vi "SVFA FFT Spectrum (Mag-Phase) (1 Ch).vi"(0 "scaled signal [EU]":waveform(dbl), 2 "window":T9=1 items=["None"=0, "Hanning"=1, "Hamming"=2, "Blackman-Harris"=3, "Exact Blackman"=4, "Blackman"=5, "Flat Top"=6, "4 Term B-Harris "=7, "7 Term B-Harris"=8, "Low Sidelobe"=9, "Force"=64, "Exponential"=65, "Blackman Nuttall"=11, "Triangle"=30, "Bartlett-Hanning"=31, "Bohman"=32, "Parzen"=33, "Welch"=34, "Kaiser"=60, "Dolph-Chebyshev"=61, "Gaussian"=62], 4 "view":T7={"dB On (T)"=TRUE, "unwrap phase (F)"=FALSE, "convert to degree (T)"=TRUE}, 5 "error in (no error)":errorcluster, 7 "averaging parameters":T8={"averaging mode"=enum."No averaging", "weighting mode"=enum."Exponential", "number of averages"=10, "linear mode"=enum."One shot"} {"number of averages" min=1 step=1}, 9 "restart averaging (F)":bool) -> (11 "averaging done":bool, 13 "averages completed":dbl, 14 "magnitude [dB EU]":cluster{"f0":dbl, "df":dbl, "magnitude":dbl[]} {"magnitude" format="%.2p"; "df" format="%.2p"; "f0" format="%.2p"}, 15 "magnitude unit label":string, 16 "phase [degrees]":cluster{"f0":dbl, "df":dbl, "phase":dbl[]} {"phase" format="%.2p"; "df" format="%.2p"; "f0" format="%.2p"}, 17 "phase unit label":string, 18 "spectrum info":T1={"channel name"="", "description"="", "x-axis units"=0, "spectral info"={"spectrum type"=enum."Power [Magnitude^2]", "linear/dB"=enum."linear", "window"=0, "window size"=0, "FFT size"=0}, "engineering units"=0, "custom label"="", "dB reference [EU]"=0.0, "peak units"=enum."rms", "weighting filter"=0, "spectral density?"=FALSE, "unit label"="", "spectrum skewed?"=FALSE, "complimentary spectrum units"=enum."none"} {"x-axis units" items=["Time (s)"=0, "Frequency-CB (Hz)"=1, "Frequency-CPB (Hz)"=1248, "Frequency-Arbitrary (Hz)"=2357, "Quefrency (s)"=2, "Revolutions (rev)"=3, "Order"=4, "Speed (RPM)"=11, "Speed (rad/s)"=21, "Index"=65535]; "weighting filter" items=["Linear", "A-weighting", "B-weighting", "C-weighting", "ITU-R 468-4", "Dolby", "CCITT", "C-message", "Wb", "Wc", "Wd", "We", "Wf", "Wh", "Wj", "Wk", "Wm", "AES17 20 kHz lowpass", "AES17 40 kHz lowpass", "AES17 20 kHz highpass", "AES17 40 kHz highpass"]; "dB reference [EU]" format="%.2f"; "engineering units" items=["custom..."=0, "V"=1, "A"=21, "C"=30, "pC"=31, "s"=32, "-"=29, "Pa"=2, "N"=20, "g"=3, "m/s^2"=4, "m/s"=5, "m"=6, "mm/s"=12, "mm"=13, "micron/s"=14, "micron"=15, "in/s^2"=7, "in/s"=8, "in"=9, "mil/s"=10, "mil"=11, "rad/s^2"=16, "rad/s"=17, "rad"=18, "deg/s^2"=26, "deg/s"=27, "deg"=28, "RPM"=22, "cycle/s^2"=23, "Hz"=24, "cycle"=25, "strain"=19]; "spectral info"."window" items=["None "=0, "Hanning"=1, "Hamming"=2, "Blackman-Harris"=3, "Exact Blackman"=4, "Blackman"=5, "Flat Top"=6, "4 Term B-Harris "=7, "7 Term B-Harris"=8, "Low Sidelobe"=9, "Force - Exponential"=10, "Gaussian"=62]}, 19 "error out":errorcluster)   [LabVIEW 2017]
doc: "Computes the Fast Fourier Transform (FFT) spectrum of <B>scaled signal [EU]</B>. This VI returns FFT results as the magnitude and phase of the FFT spectrum. Wire data to the <B>scaled signal [EU]</B> input to determine the polymorphic instance to use or manually select the instance."
uses:
  <vilib>/addons/_NISVFA/_Shared subVIs/Controls/svc_Window.ctl
  <vilib>/addons/_NISVFA/_Shared subVIs/Controls/svc_Spectrum Info.ctl
  <vilib>/addons/_NISVFA/_Shared subVIs/Controls/svc_X-Axis Units.ctl
  <vilib>/addons/_NISVFA/_Shared subVIs/Controls/svc_Spectrum Type.ctl
  <vilib>/addons/_NISVFA/_Shared subVIs/Controls/svc_Engineering Units Text Ring.ctl
  <vilib>/addons/_NISVFA/_Shared subVIs/Controls/svc_Weighting Filter Text Ring.ctl
  <vilib>/addons/_NISVFA/_Shared subVIs/Controls/svc_Complimentary Spectrum Units.ctl
  <vilib>/Analysis/2dsp.llb/Real FFT.vi
  <vilib>/Analysis/2dsp.llb/Power Spectrum (DBL).vi
  <vilib>/addons/_NISVFA/_Shared subVIs/Spectrum Averaging/svfa_No Average Array (complex).vi
  <vilib>/addons/_NISVFA/_Shared subVIs/Spectrum Averaging/svfa_Average Array (complex).vi
  <vilib>/addons/_NISVFA/_Shared subVIs/Spectrum Averaging/svfa_No Average Array (real).vi
  <vilib>/addons/_NISVFA/_Shared subVIs/Spectrum Averaging/svfa_Average Array (real).vi
  <vilib>/addons/_NISVFA/_Shared subVIs/Spectrum Averaging/svfa_Peak Hold Array.vi
  <vilib>/addons/_NISVFA/_Shared subVIs/Windowing/svfa_Scaled Time Domain Window (Array).vi
  <vilib>/addons/_NISVFA/_Shared subVIs/Common/svc_Get SV Channel Info.vi
  <vilib>/addons/_NISVFA/_Shared subVIs/Common/svc_Spectrum Units.vi
  <vilib>/Analysis/4window.llb/Force Window.vi
  <vilib>/Analysis/4window.llb/Force Window (DBL).vi
  <vilib>/Analysis/4window.llb/Exponential Window.vi
  <vilib>/Analysis/4window.llb/Exponential Window (DBL).vi
  <vilib>/addons/_NISVFA/_Shared subVIs/Common/svc_Get Weighting Enum and Labels.vi
  <vilib>/addons/_NISVFA/_Shared subVIs/Common/svc_Unit Label Lexical Class.vi
  <vilib>/addons/_NISVFA/_Shared subVIs/Common/svc_Engineering Units to Unit Label.vi
  <vilib>/addons/_NISVFA/_Shared subVIs/Common/svc_Format Value (DBL).vi
  <vilib>/addons/_NISVFA/_Shared subVIs/Common/svc_Channel Info to Spectrum Info.vi
  <vilib>/addons/_NISVFA/_Shared subVIs/Common/svc_Unit Label to Engineering Units.vi
  <vilib>/Utility/error.llb/Error Cluster From Error Code.vi
  <vilib>/Analysis/0measdsp.llb/Scaled Time Domain Window.vi
  <vilib>/Analysis/0measdsp.llb/Scaled Time Domain Window (DBL).vi
  <vilib>/addons/_NISVFA/_Spectrum Processing/subVIs/svfa_Spectrum Info Window to windowTd Type Def.vi
  <vilib>/addons/_NISVFA/_Shared subVIs/Common/svc_Window Parameters.vi
  <vilib>/addons/_NISVFA/_Shared subVIs/Common/svc_Get Window Info.vi
  <vilib>/Analysis/NI_AALPro.lvlib
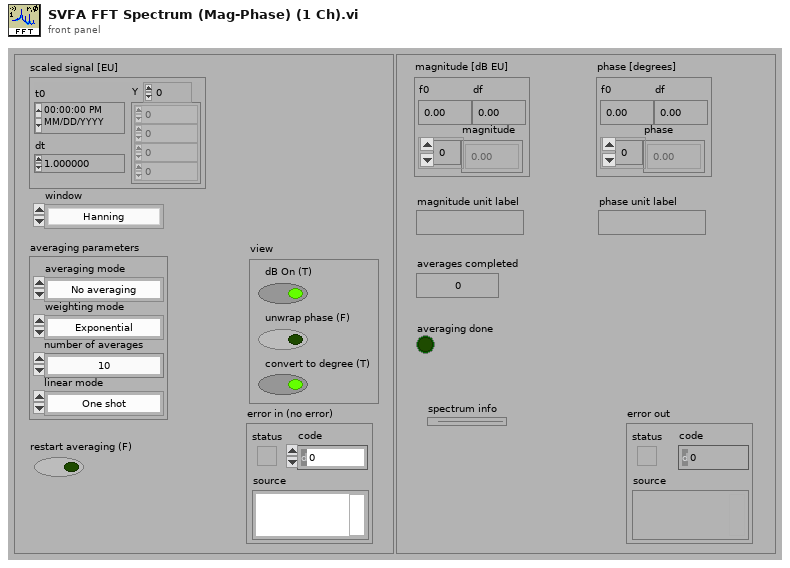
[diagram p1: front panel]
types:
  T1 = typedef "svc_Spectrum Info.ctl" = cluster{"channel name":string, "description":string, "x-axis units":T2, "spectral info":cluster{"spectrum type":T3, "linear/dB":enum16{"linear", "dB"}, "window":u16, "window size":i32, "FFT size":i32}, "engineering units":T4, "custom label":string, "dB reference [EU]":dbl, "peak units":enum16{"rms", "peak", "peak-peak"}, "weighting filter":T5, "spectral density?":bool, "unit label":string, "spectrum skewed?":bool, "complimentary spectrum units":T6}
  T2 = typedef "svc_X-Axis Units.ctl" = u16
  T3 = typedef "svc_Spectrum Type.ctl" = enum16{"FFT Spectrum [complex]", "Amplitude [Magnitude]", "Power [Magnitude^2]", "Cross Spectrum [complex]", "Frequency Response [Complex]"}
  T4 = typedef "svc_Engineering Units Text Ring.ctl" = u16
  T5 = typedef "svc_Weighting Filter Text Ring.ctl" = u16
  T6 = typedef "svc_Complimentary Spectrum Units.ctl" = enum16{"none", "radians", "degrees", "cycles", "imaginary"}
  T7 = cluster{"dB On (T)":bool, "unwrap phase (F)":bool, "convert to degree (T)":bool}
  T8 = cluster{"averaging mode":enum16{"No averaging", "Vector averaging", "RMS averaging", "Peak hold"}, "weighting mode":enum16{"Linear", "Exponential"}, "number of averages":u32, "linear mode":enum16{"One shot", "Auto restart"}}
  T9 = typedef "svc_Window.ctl" = u32
  T10 = cluster{"f0":dbl, "df":dbl, "complex spectrum":cdb[]}
  T11 = enum16{"Restart processing", "Continue processing", "Skip processing"}
  T12 = enum16{"No averaging", "Vector averaging", "RMS averaging", "Peak hold"}
  T13 = cluster{"complex FFT":cdb[], "real FFT":dbl[], "f0":dbl, "df":dbl, "averages completed":dbl, "averaging parameters":cluster{"averaging mode":enum16{"No averaging", "Vector averaging", "RMS averaging", "Peak hold"}, "weighting mode":enum16{"Linear", "Exponential"}, "number of averages":u32, "linear mode":enum16{"One shot", "Auto restart"}}}
  T14 = cluster{"complex FFT":cdb[], "Mag/Real FFT":dbl[], "f0":dbl, "df":dbl, "averages completed":dbl, "averaging parameters":cluster{"averaging mode":enum16{"No averaging", "Vector averaging", "RMS averaging", "Peak hold"}, "weighting mode":enum16{"Linear", "Exponential"}, "number of averages":u32, "linear mode":enum16{"One shot", "Auto restart"}}}
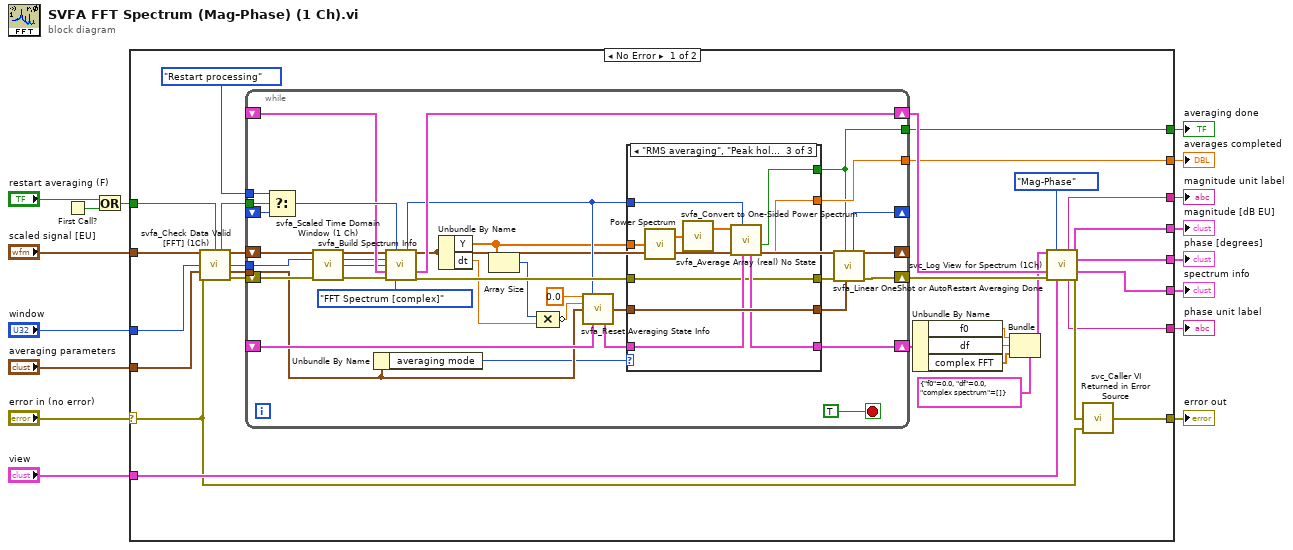
[diagram p0: block diagram]
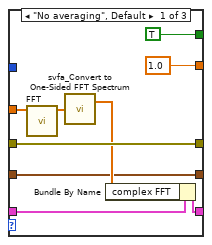
[diagram p2: hidden frame]
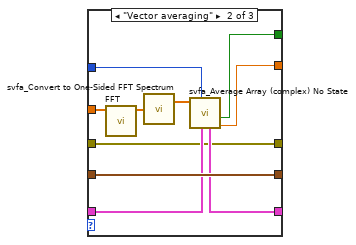
[diagram p3: hidden frame]
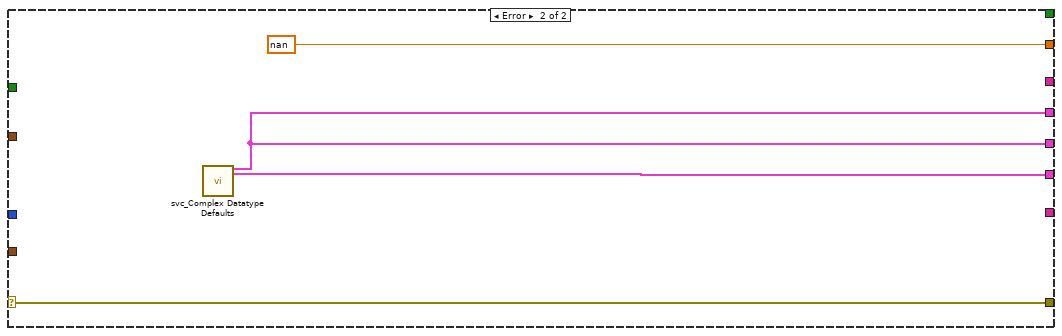
[diagram p4: hidden frame]
diagram:
  n1 = First Call?() -> (First Call?: T/F=w3:bool)
  n2 = Or(x="restart averaging (F)", y=w3) -> (x .or. y?=w1:bool)
  n3 = case shown="No Error" "error in (no error)" {
    selector: "error in (no error)" -> [w18 w114]
    tunnel: [w21 w111] -> w4
    tunnel: "window" -> [w29 _]
    tunnel: "averaging parameters" -> [w30 _]
    tunnel: "view" -> [w28 _]
    tunnel: [w20 w114] -> w16
    tunnel: [w25 _] -> w15
    tunnel: [w26 _] -> w14
    tunnel: "scaled signal [EU]" -> [w31 _]
    tunnel: w1 -> [w17 _]
    tunnel: [w23 nan ("averages completed")] -> w9
    tunnel: [w24 _] -> w8
    tunnel: [w19 w112] -> w6
    tunnel: [w22 w111] -> w5
    frame No Error {
      n4 = call <vilib>:"svfa_Check Data Valid [FFT] (1Ch).vi"("signal in [X]"=w31, "restart averaging (F)"=w17, "window"=w29, "averaging parameters"=w30, "error in (no error)"=w18) -> ("restart averaging"=w39:bool, "dup signal in [X]"=w43:waveform(dbl), "dup window"=w42:T9, "dup averaging parameters"=w41:T8, "error out"=w40:errorcluster)  [unwired: 6 in]
      n5 = while {
        shift-left: _ -> [w73]
        shift-right: [w74] -> w44
        tunnel: w39 -> [w71]
        tunnel: [w79] -> w24
        tunnel: [w81] -> w23
        shift-right: [w80] -> _
        shift-left: _ -> [w70]
        shift-right: [w72] -> w37
        shift-left: _ -> [w68]
        tunnel: T11."Restart processing" ("t") -> [w67]
        tunnel: w41 -> [w66]
        tunnel: w42 -> [w65]
        shift-right: [w47] -> _
        shift-left: w43 -> [w78]
        shift-right: [w76] -> w36
        shift-left: w40 -> [w77]
        stop <- TRUE stop-if-true
        n6 = Select(t=w67, s=w71, f=w70) -> (s? t:f=w69:T11)
        n7 = call <vilib>:"svfa_Scaled Time Domain Window (1 Ch).vi"("Signal in [X]"=w78, "window"=w65, "error in"=w77) -> ("Windowed Waveform"=w61:waveform(dbl), "dup window"=w59:T9, "window length"=w51:i32, "error out"=w63:errorcluster)  [unwired: 7 in, 2 out]
        n8 = Unbundle By Name(w66) -> ("averaging mode"=w64:T12)
        n9 = call <vilib>:"svfa_Build Spectrum Info.vi"("scaled signal [EU]"=w61, "processing control"=w69, "window"=w59, "window size"=w51, "spectrum info in"=w68, "error in (no error)"=w63, "spectrum type"=svc_Spectrum_Type."FFT Spectrum [complex]") -> ("dup processing control"=w57:T11, "dup scaled signal [EU]"=w47:waveform(dbl), "spectrum info out"=w72:T1, "error out"=w62:errorcluster)  [unwired: 5 in]
        n10 = Unbundle By Name ("Get Waveform Components")(w47) -> ("Y"=w50:dbl[], "dt"=w52:dbl)
        n11 = Array Size(array=w50) -> (size(s)=w49:i32)
        n12 = Compound Arithmetic op=MULTIPLY(w49, w52) -> (invert w48:dbl)
        n13 = call <vilib>:"svfa_Reset Averaging State Info.vi"("f0"=0.0, "processing control"=w57, "df"=w48, "averaging parameters"=w66, "averaging state info in"=w73) -> ("dup averaging parameters"=w55:T8, "averaging state info out"=w56:T13)  [unwired: 9 in]
        n14 = case shown="\"RMS averaging\", \"Peak hold\"" w64 {
          tunnel: [w88 w93 w101] -> w60
          tunnel: [TRUE ("averaging done") w92 w103] -> w79
          tunnel: [1.0 ("averages completed") w91 w102] -> w81
          tunnel: w50 -> [w86 w99 w109]
          tunnel: w62 -> [w88 w93 w101]
          tunnel: w57 -> [_ w94 w106]
          tunnel: w55 -> [w82 w97 w107]
          tunnel: [w84 w95 w104] -> w74
          tunnel: w56 -> [w85 w96 w105]
          tunnel: [w82 w97 w107] -> w54
          frame "No averaging", Default {
            n15 = call-poly <vilib>:"FFT.vi"("X"=w86) -> ("FFT {X}"=w87:cdb[])  [unwired: 9 in, 1 out]
            n16 = call <vilib>:"svfa_Convert to One-Sided FFT Spectrum.vi"("two-sided FFT spectrum"=w87) -> ("one-sided FFT spectrum"=w83:cdb[])  [unwired: 1 out]
            n17 = Bundle By Name(cluster=w85, "complex FFT"=w83) -> (w84:T13)
          }
          frame "Vector averaging" {
            n18 = call-poly <vilib>:"FFT.vi"("X"=w99) -> ("FFT {X}"=w100:cdb[])  [unwired: 9 in, 1 out]
            n19 = call <vilib>:"svfa_Convert to One-Sided FFT Spectrum.vi"("two-sided FFT spectrum"=w100) -> ("one-sided FFT spectrum"=w98:cdb[])  [unwired: 1 out]
            n20 = call <vilib>:"svfa_Average Array (complex) No State.vi"("averaging state info in"=w96, "processing control"=w94, "array"=w98) -> ("averages completed"=w91:dbl, "averaging done"=w92:bool, "averaging state info out"=w95:T14)  [unwired: 5 in, 1 out]
          }
          frame "RMS averaging", "Peak hold" {
            n21 = call-poly <vilib>:"Power Spectrum.vi"("X"=w109) -> ("Power Spectrum"=w110:dbl[])  [unwired: 1 out]
            n22 = call <vilib>:"svfa_Convert to One-Sided Power Spectrum.vi"("two-sided power spectrum"=w110) -> ("one-sided power spectrum"=w108:dbl[])  [unwired: 1 out]
            n23 = call <vilib>:"svfa_Average Array (real) No State.vi"("averaging state info in"=w105, "processing control"=w106, "array"=w108) -> ("averages completed"=w102:dbl, "averaging done"=w103:bool, "averaging state info out"=w104:T14)  [unwired: 5 in, 1 out]
          }
        }
        n24 = call <vilib>:"svfa_Linear OneShot or AutoRestart Averaging Done.vi"("averaging parameters"=w54, "averaging done"=w79, "error in (no error)"=w60) -> ("error out"=w76:errorcluster, "processing control"=w80:T11)  [unwired: 7 in]
      }
      n25 = Unbundle By Name(w44) -> ("f0"=w35:dbl, "df"=w34:dbl, "complex FFT"=w33:cdb[])
      n26 = Bundle(cluster=T10 {"f0"=0.0, "df"=0.0, "complex spectrum"=[]} ("complex spectrum response"), "f0"=w35, "df"=w34, "complex spectrum"=w33) -> (w32:T10)
      n27 = call <vilib>:"svc_Log View for Spectrum (1Ch).vi"("complex spectrum"=w32, "View"=enum16{"Mag-Phase", "Real-Imaginary"}."Mag-Phase", "spectrum info in"=w37, "error in (no error)"=w36, "view"=w28) -> ("unit label [mag or real]"=w25:string, "magnitude or real"=w22:cluster{"f0":dbl, "df":dbl, dbl[]}, "phase or imag"=w21:cluster{"f0":dbl, "df":dbl, dbl[]}, "spectrum info out"=w19:T1, "unit label [phase or imag]"=w26:string, "error out"=w46:errorcluster)  [unwired: 5 in]
      n28 = call <vilib>:"svc_Caller VI Returned in Error Source.vi"("warning input to caller"=w18, "error in (no error)"=w46) -> ("error out"=w20:errorcluster)  [unwired: 3 in]
    }
    frame Error {
      n29 = call <vilib>:"svc_Complex Datatype Defaults.vi"() -> ("empty spectrum"=w111:cluster{"f0":dbl, "df":dbl, "magnitude":dbl[]}, "dead spectrum info"=w112:T1)  [unwired: 11 in, 7 out]
    }
  }
  "error out" <- w16
  "magnitude [dB EU]" <- w5
  "phase [degrees]" <- w4
  "magnitude unit label" <- w15
  "phase unit label" <- w14
  "averages completed" <- w9
  "averaging done" <- w8
  "spectrum info" <- w6
